vi "UI_Log_In.vi"() -> ()   [LabVIEW 2014]
uses:
  Terminal_Global_User_name.vi
panel:
  in  "登录":bool
  in  "取消":bool
  in  "身份":u16(ring) items=["管理员", "普通用户"]
  in  "密码":string="123"
  in  "用户名":string="管理员1"
  # "欢迎使用\n\n                           轴承测试系统"
  # "版本:1.0\n\n\n  (c) 2015                  版权所有 *****************"
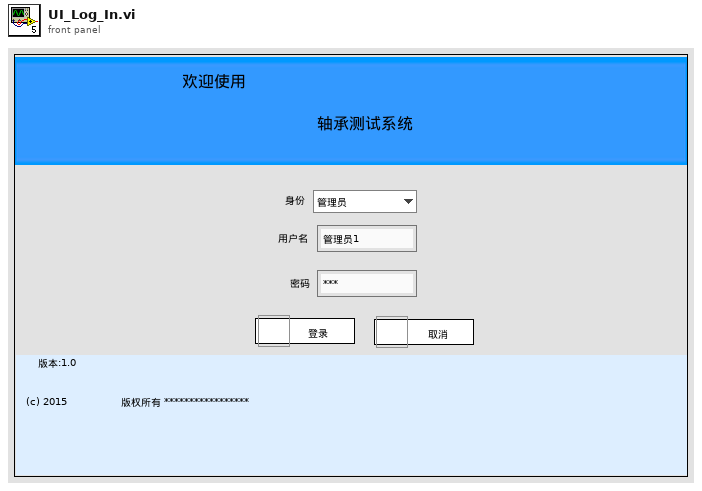
[diagram p1: front panel]
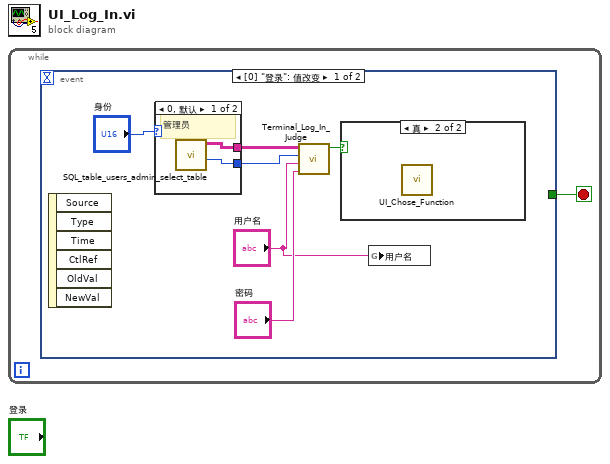
[diagram p0: block diagram]
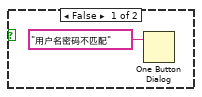
[diagram p2: hidden frame]
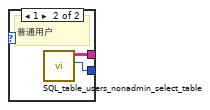
[diagram p3: hidden frame]
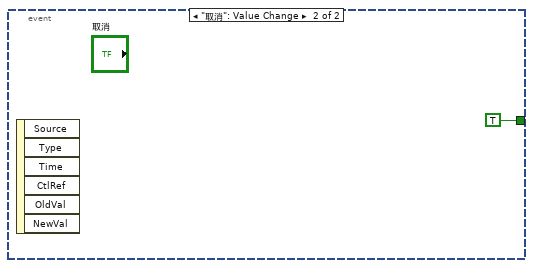
[diagram p4: hidden frame]
diagram:
  n1 = while {
    stop <- w1 stop-if-true
    n2 = event shown="[0] \"登录\": 值改变" {
      selector: _ -> [_ _]
      dyn-events: _ -> [_ _]
      timeout: _ -> [_ _]
      tunnel: [_ TRUE] -> w1
      event "登录": Value Change {
        n3 = event-data() -> ()  [unwired: 1 in, 6 out]
        n4 = case shown="0, 默认" "身份" {
          tunnel: [w10 w12] -> w6
          tunnel: [w9 w11] -> w5
          frame 0, Default {
            # "管理员"
            n5 = call "SQL_table_users_admin_select_table.vi"() -> ("管理员个数"=w9:i32, "管理员信息"=w10:string[][])  [unwired: 9 in, 1 out]
          }
          frame 1 {
            # "普通用户"
            n6 = call "SQL_table_users_nonadmin_select_table.vi"() -> ("普通用户个数"=w11:i32, "普通用户信息"=w12:string[][])  [unwired: 9 in, 1 out]
          }
        }
        n7 = call "Terminal_Log_In_Judge.vi"("密码"="密码", "用户名"="用户名", "用户个数"=w5, "用户名密码信息"=w6) -> ("用户名密码匹配"=w3:bool)  [unwired: 7 in]
        n8 = case shown="真" w3 {
          frame False {
            n9 = One Button Dialog(message="用户名密码不匹配") -> ()  [unwired: 1 in, 1 out]
          }
          frame True {
            n10 = call "UI_Chose_Function.vi"() -> ()  [unwired: 12 in]
          }
        }
        n11 = global write "Terminal_Global_User_name.vi" "用户名"("用户名") -> ()
      }
      event "取消": Value Change {
        n12 = event-data() -> ()  [unwired: 1 in, 6 out]
      }
    }
  }
